vi "quintofor.vi"() -> ()   [LabVIEW 2012]
panel:
  in  "stop":bool
  out "Waveform Graph":dbl[](graph)
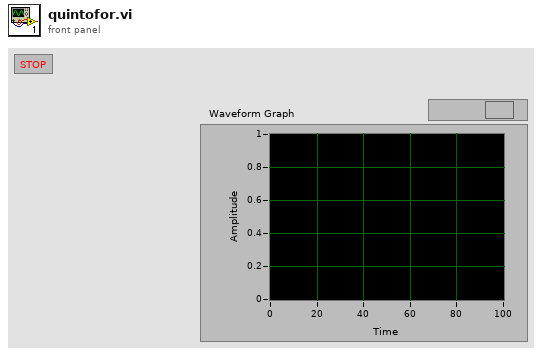
[diagram p1: front panel]
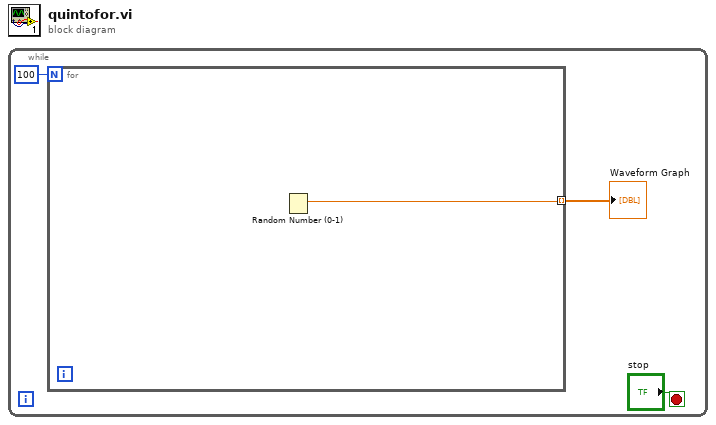
[diagram p0: block diagram]
diagram:
  n1 = while {
    stop <- "stop" stop-if-true
    n2 = for {
      N: 100 -> [_]
      tunnel: [w4] -> w2 mode=indexing
      n3 = Random Number (0-1)() -> (number: 0 to 1=w4:dbl)
    }
    "Waveform Graph" <- w2
  }
